vi "外控留样模式参数.vi"() -> ()   [LabVIEW 2016, in "超标留样集成.lvlib" / "ESTD1200.lvlib"]
uses:
  ESTD1200.lvlib
  <vilib>/Utility/miscctls.llb/LVPointTypeDef.ctl
panel:
  out "读取更新":bool
  in  "返回":bool
  in  "模拟设置":bool
  in  "每瓶次数：":dbl
  in  "平行样：":dbl
  in  "每次留样：":dbl
  in  "留样瓶数：":dbl
  in  "当前瓶号：":dbl
  # "在该画面下，可设置该模式下的采样参数，包括当前瓶号、平行样、留样瓶数、每瓶次数和每次留样量。"
  # "mL"
  # "mg/L"
  # "COD\n模拟\n设置"
  # "mg/L"
  # "mg/L"
  # "mg/L"
  # "mg/L"
  # "氨氮\n模拟\n设置"
  # "mg/L"
  # "mg/L"
  # "mg/L"
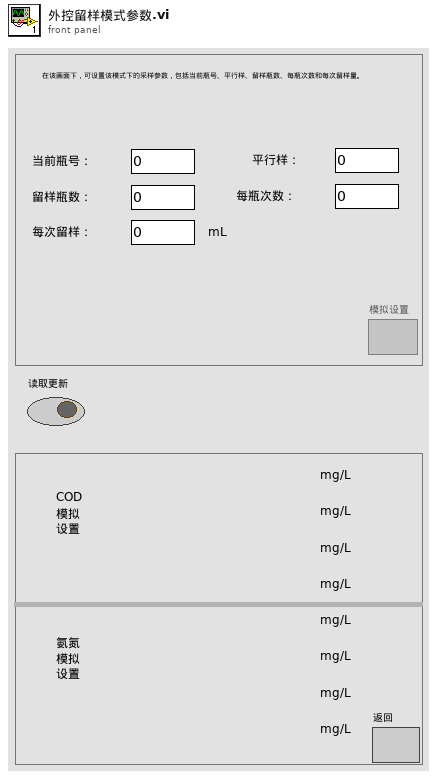
[diagram p1: front panel]
types:
  T1 = typedef "LVPointTypeDef.ctl" = cluster{"Horizontal":i16, "Vertical":i16}
  T2 = cluster{"当前瓶号：":dbl, "平行样：":dbl, "留样瓶数：":dbl, "每瓶次数：":dbl, "每次留样：":dbl}
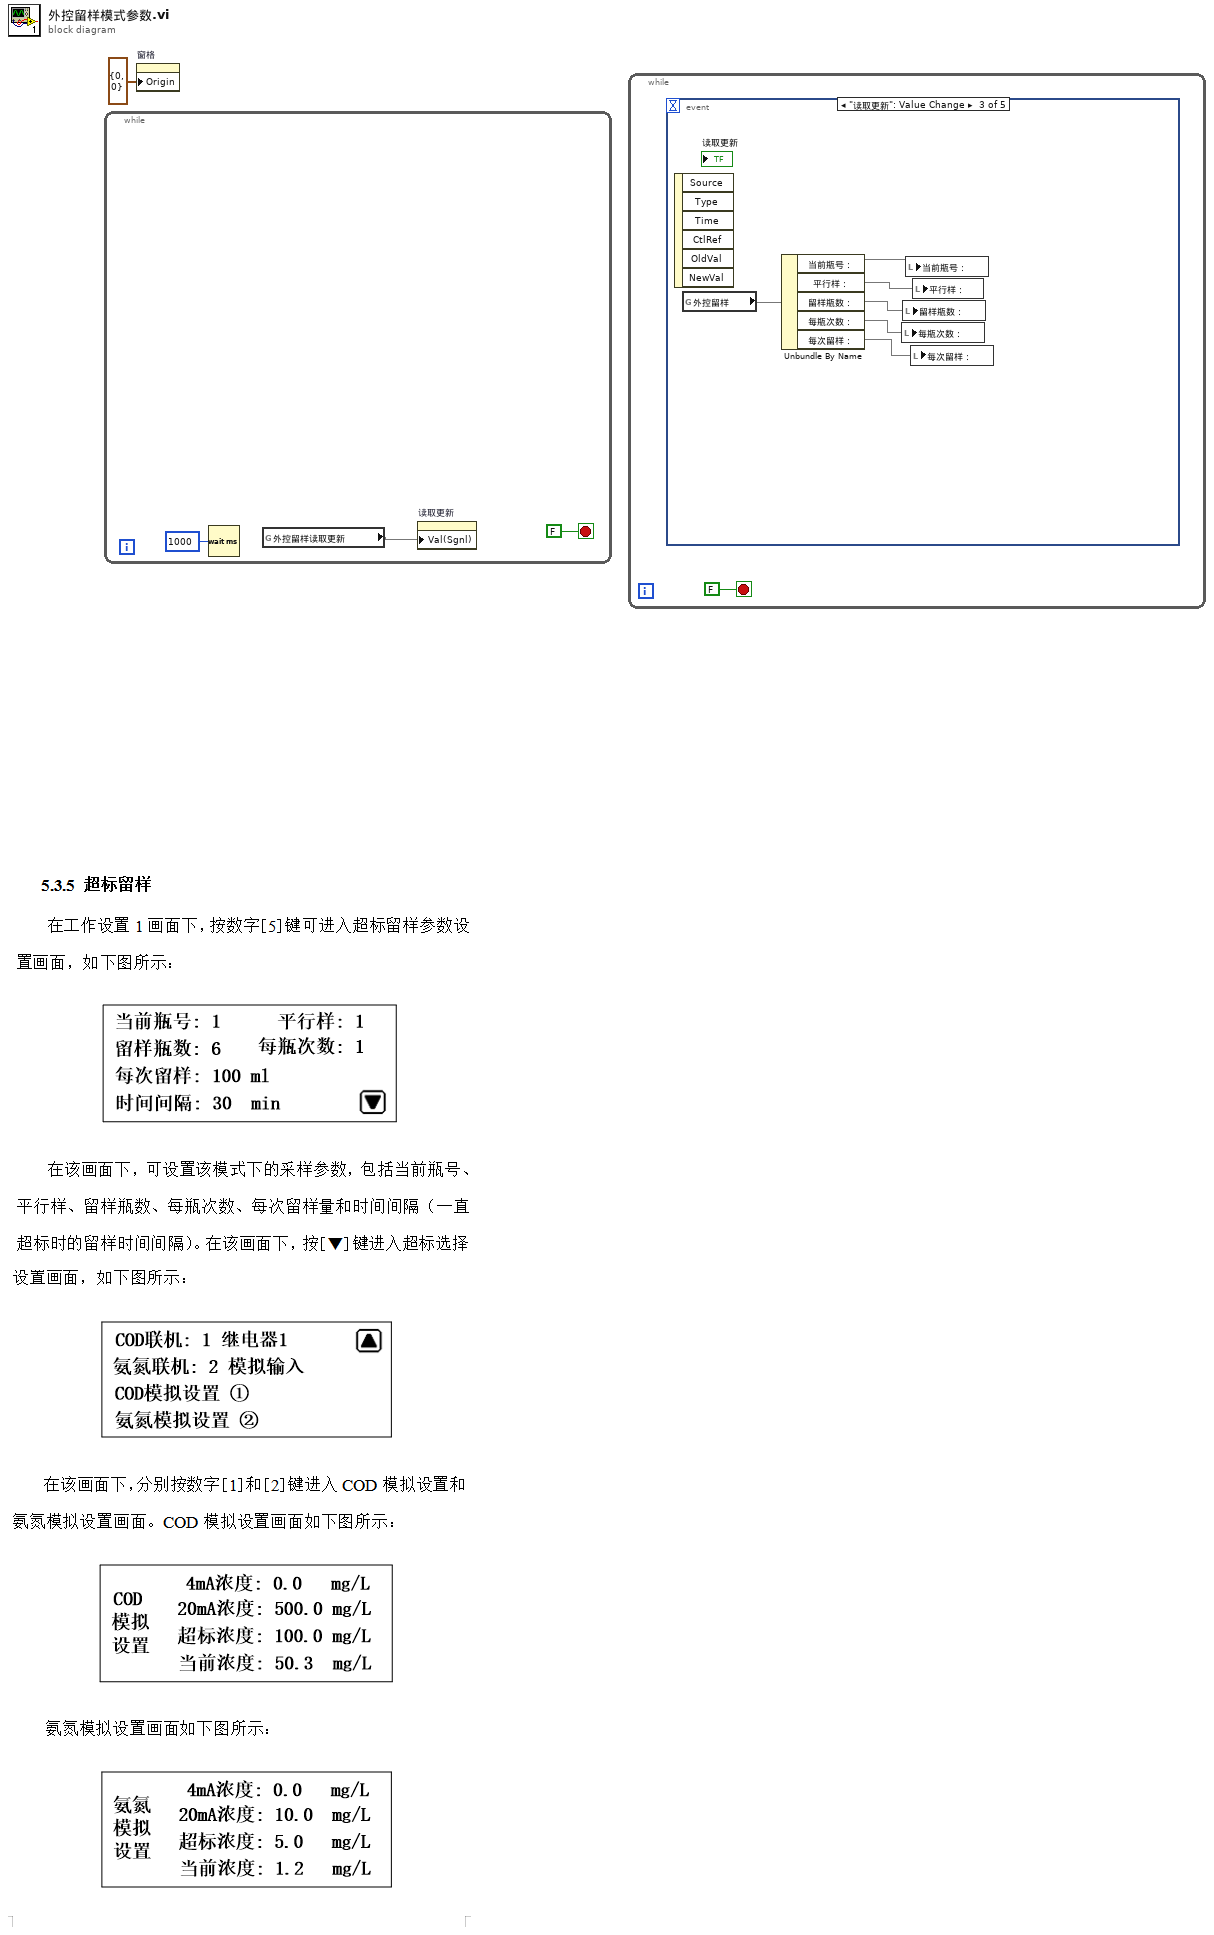
[diagram p0: block diagram]
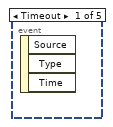
[diagram p2: hidden frame]
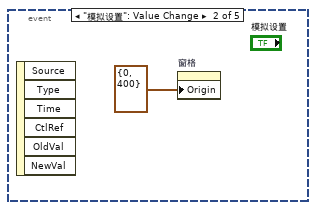
[diagram p3: hidden frame]
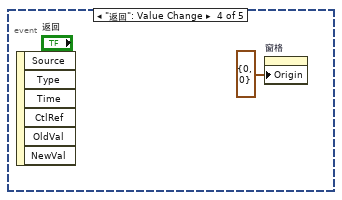
[diagram p4: hidden frame]
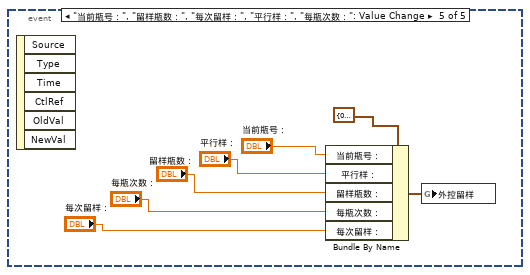
[diagram p5: hidden frame]
diagram:
  n1 = while {
    stop <- FALSE stop-if-true
    n2 = Wait (ms)(milliseconds to wait=u32 1000 ("等待时间（毫秒）")) -> ()  [unwired: 1 out]
    n3 = global read "超标留样全局.vi" "外控留样读取更新"() -> (w2)
    n4 = property on="读取更新" class="Bool (strict)"("Val(Sgnl)"=w2) -> ()  [unwired: 2 in, 2 out]
  }
  n5 = property on="窗格" class="Pane"("Origin"=T1 {"Horizontal"=0, "Vertical"=0} ("原点")) -> ()  [unwired: 2 in, 2 out]
  n6 = while {
    stop <- FALSE stop-if-true
    n7 = event shown="[2] \"读取更新\": Value Change" {
      selector: _ -> [_ _ _ _ _]
      dyn-events: _ -> [_ _ _ _ _]
      timeout: _ -> [_ _ _ _ _]
      event Timeout {
        n8 = event-data() -> ()  [unwired: 1 in, 3 out]
      }
      event "模拟设置": Value Change {
        n9 = event-data() -> ()  [unwired: 1 in, 6 out]
        n10 = property on="窗格" class="Pane"("Origin"=T1 {"Horizontal"=0, "Vertical"=400} ("原点")) -> ()  [unwired: 2 in, 2 out]
      }
      event "读取更新": Value Change {
        n11 = event-data() -> ()  [unwired: 1 in, 6 out]
        n12 = global read "超标留样全局.vi" "外控留样"() -> (w12)
        n13 = Unbundle By Name(w12) -> ("当前瓶号："=w11, "平行样："=w10, "留样瓶数："=w9, "每瓶次数："=w8, "每次留样："=w7)
        n14 = local write "每瓶次数："(w8) -> ()
        n15 = local write "留样瓶数："(w9) -> ()
        n16 = local write "当前瓶号："(w11) -> ()
        n17 = local write "每次留样："(w7) -> ()
        n18 = local write "平行样："(w10) -> ()
      }
      event "返回": Value Change {
        n19 = event-data() -> ()  [unwired: 1 in, 6 out]
        n20 = property on="窗格" class="Pane"("Origin"=T1 {"Horizontal"=0, "Vertical"=0} ("原点")) -> ()  [unwired: 2 in, 2 out]
      }
      event "当前瓶号：", "留样瓶数：", "每次留样：", "平行样：", "每瓶次数：": Value Change {
        n21 = event-data() -> ()  [unwired: 1 in, 6 out]
        n22 = Bundle By Name(cluster=T2 {"当前瓶号："=0.0, "平行样："=0.0, "留样瓶数："=0.0, "每瓶次数："=0.0, "每次留样："=0.0} ("外控留样"), "当前瓶号："="当前瓶号：", "平行样："="平行样：", "留样瓶数："="留样瓶数：", "每瓶次数："="每瓶次数：", "每次留样："="每次留样：") -> (w14:T2)
        n23 = global write "超标留样全局.vi" "外控留样"(w14) -> ()
      }
    }
  }
